vi "Test DMM.vi"() -> ()   [LabVIEW 2020, in "Digital Multimeter.lvclass"]
uses:
  Digital Multimeter.lvclass
  HP 3457A/HP 3457A.lvclass
  C:/Sandbox/Git_Sandbox/WiSpry Test Framework source code (LV20)/WiSpry Test Framework/Instruments/Instrument.lvclass
  Instrument.lvclass/Instrument.ctl
  Instrument.lvclass
panel:
  out "Unit":string
  out "Measure":dbl
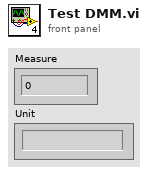
[diagram p1: front panel]
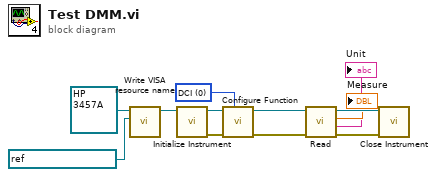
[diagram p0: block diagram]
diagram:
  w3 = u16 0 items=["DCI", "DCV"] ("Function")
  n1 = call "Write VISA resource name.vi"("VISA resource name"=refnum<visa-resource-name> "GPIB0::4::INSTR", "Instrument in"=refnum<class "HP 3457A.lvclass"> refnum ("HP 3457A.lvclass")) -> ("Instrument out"=w11:refnum<class "HP 3457A.lvclass">)  [unwired: 9 in]
  n2 = call-dynamic "Initialize Instrument.vi"("HP 3457A in"=w11) -> ("error out"=w9:errorcluster, "HP 3457A out"=w10:refnum<class "HP 3457A.lvclass">)  [unwired: 9 in]
  n3 = call-dynamic "Configure Function.vi"("Function"=w3, "error in (no error)"=w9, "HP 3457A in"=w10) -> ("error out"=w6:errorcluster, "HP 3457A out"=w7:refnum<class "HP 3457A.lvclass">)  [unwired: 7 in]
  n4 = call-dynamic "Read.vi"("error in (no error)"=w6, "HP 3457A in"=w7) -> ("error out"=w4:errorcluster, "Unit"=→"Unit":string, "Measure"=→"Measure":dbl, "HP 3457A out"=w5:refnum<class "HP 3457A.lvclass">)  [unwired: 5 in, 1 out]
  n5 = call-dynamic "Close Instrument.vi"("error in (no error)"=w4, "Instrument in"=w5) -> ()  [unwired: 8 in, 2 out]
